vi "FPGAmain_5782_Fast_PID_v2.vi"() -> ()   [LabVIEW 2013]
uses:
  FPGA/DataMode.ctl
  FPGA/Input_5782/5782_states.ctl
  <vilib>/Platform/TimedLoop/XDataNode/timing_clust.ctl
  <vilib>/Platform/TimedLoop/XDataNode/nitl_modes.ctl
  <vilib>/Platform/TimedLoop/XDataNode/wakeup.ctl
  <vilib>/rvi/Emulation/niFpgaSctlEmulationGetInTimedLoop.vi
  <vilib>/rvi/Emulation/niFpgaEmulationReportErrorSimple.vi
  <vilib>/rvi/Emulation/niFpgaGetClockAttributes.vi
  <vilib>/rvi/eio/common/nirviEmuTemplateMethod_errors.vi
  <vilib>/rvi/Emulation/niFpgaCriticalErrorInLSC.vi
  <vilib>/rvi/DataTransferAndStorage/Register/Emulation/niFpgaRegisterEmulationFpgaImpl.vi
  <instcachedir>/0/niFpgaRegisterEmulationFpgaImpl_DCF4BC0110594B98B44A971D60CEEC4D.lvgen/niFpgaRegisterEmulationFpgaImpl_DCF4BC0110594B98B44A971D60CEEC4D_009.vi
  <vilib>/rvi/DataTransferAndStorage/Container/Common/niFpgaContainerGetUniqueNameForEmu.vi
  <vilib>/rvi/FIFO/Fifo_Resource/nirvififoEmulationReadFpgaImpl.vi
  <vilib>/rvi/interface/RandomDataEmulation/nirviRandomDataMultiElementFPGAFIFO.vi
  <instcachedir>/0/nirviRandomDataMultiElementFPGAFIFO_F2B80EDE0D7944A08478D8D26097D4DB.lvgen/nirviRandomDataMultiElementFPGAFIFO_F2B80EDE0D7944A08478D8D26097D4DB_005.vi
  <vilib>/rvi/interface/RandomDataEmulation/niFpgaRandomDataHandleErrors.vi
  <instcachedir>/0/niFpgaRegisterEmulationFpgaImpl_DCF4BC0110594B98B44A971D60CEEC4D.lvgen/niFpgaRegisterEmulationFpgaImpl_DCF4BC0110594B98B44A971D60CEEC4D_013.vi
  <vilib>/rvi/interface/RandomDataEmulation/nirviRandomDataFPGAFIFO.vi
  <instcachedir>/0/niFpgaRegisterEmulationFpgaImpl_DCF4BC0110594B98B44A971D60CEEC4D.lvgen/niFpgaRegisterEmulationFpgaImpl_DCF4BC0110594B98B44A971D60CEEC4D_003.vi
  <vilib>/rvi/FIFO/Fifo_Resource/nirvififoEmulationWriteFpgaImpl.vi
  <instcachedir>/0/niFpgaRegisterEmulationFpgaImpl_DCF4BC0110594B98B44A971D60CEEC4D.lvgen/niFpgaRegisterEmulationFpgaImpl_DCF4BC0110594B98B44A971D60CEEC4D_011.vi
  <instcachedir>/0/niFpgaRegisterEmulationFpgaImpl_DCF4BC0110594B98B44A971D60CEEC4D.lvgen/niFpgaRegisterEmulationFpgaImpl_DCF4BC0110594B98B44A971D60CEEC4D_012.vi
  <instcachedir>/0/niFpgaRegisterEmulationFpgaImpl_DCF4BC0110594B98B44A971D60CEEC4D.lvgen/niFpgaRegisterEmulationFpgaImpl_DCF4BC0110594B98B44A971D60CEEC4D_007.vi
  <instcachedir>/0/niFpgaRegisterEmulationFpgaImpl_DCF4BC0110594B98B44A971D60CEEC4D.lvgen/niFpgaRegisterEmulationFpgaImpl_DCF4BC0110594B98B44A971D60CEEC4D_008.vi
  <instcachedir>/0/niFpgaRegisterEmulationFpgaImpl_DCF4BC0110594B98B44A971D60CEEC4D.lvgen/niFpgaRegisterEmulationFpgaImpl_DCF4BC0110594B98B44A971D60CEEC4D_021.vi
  <instcachedir>/0/niFpgaRegisterEmulationFpgaImpl_DCF4BC0110594B98B44A971D60CEEC4D.lvgen/niFpgaRegisterEmulationFpgaImpl_DCF4BC0110594B98B44A971D60CEEC4D_020.vi
  <vilib>/Platform/TimedLoop/XDataNode/XDataNode.xnode
  <vilib>/eio/EIONode/EIONode.xnode
  <vilib>/rvi/DataTransferAndStorage/Container/XNode/niFpgaContainer.xnode
  <vilib>/rvi/DataTransferAndStorage/Register/Emulation/niFpgaRegisterEmulation.vi
  <vilib>/rvi/FIFO/Fifo_Resource/nirvififoEmulationRead.vi
  <vilib>/rvi/interface/RandomDataEmulation/nirviRandomDataFpgaMultiElementTemplate.vi
  <vilib>/rvi/interface/RandomDataEmulation/nirviRandomDataFpgaReadWriteTemplate.vi
  <vilib>/rvi/FIFO/Fifo_Resource/nirvififoEmulationWrite.vi
  <vilib>/Platform/TimedLoop/XDataNode/XDNodeRunTimeDep.lvlib
panel:
  in  "IO Module\\AO Data Sync":bool=TRUE
  in  "IO Module\\SPI Write Data":u16
  out "IO Module\\SPI Read Data":u8
  in  "IO Module\\SPI Read":bool
  in  "IO Module\\SPI Write":bool
  in  "IO Module\\SPI Address":u16
  in  "IO Module\\SPI Device":u8
  out "IO Module\\SPI Idle":bool
  in  "AM phase":fxp<+,64,64>
  in  "delay phase":fxp<+,64,64>
  in  "User Command Commit":bool
  in  "User Command":u8
  out "User Command Idle":bool
  out "User Command Status":u8
  in  "User Data 0":u8
  in  "User Data 1":u8
  out "PLL Locked":bool
  out "User Error":bool
  out "Configured?":bool
  in  "Continuous":bool
  in  "5782 record length":u16=4000 caption="Samples Per Trigger" min=1 step=1
  in  "Trigger Acquisition":bool
  out "IO Module\\Trigger Input":bool
  in  "Downsample":fxp<+,8,8>=1.0
  in  "new coeffs":bool
  in  "FIR coeffs":fxp<+/-,18,18>[](array[numeric])
  in  "CIC Gain":fxp<+/-,32,1>=0.00390625 format="%#_32g"
  in  "Acquisition running":bool
  in  "Phase output":fxp<+,64,64>[](array[numeric])=[0.0, 0.0, 0.0, 0.0]
  in  "Simulated phase 5782":fxp<+,64,64>[](array[numeric])=[0.0, 0.0]
  in  "Mode":T1
  in  "Phase 5782":fxp<+,64,64>[](array[numeric])=[0.0, 0.0]
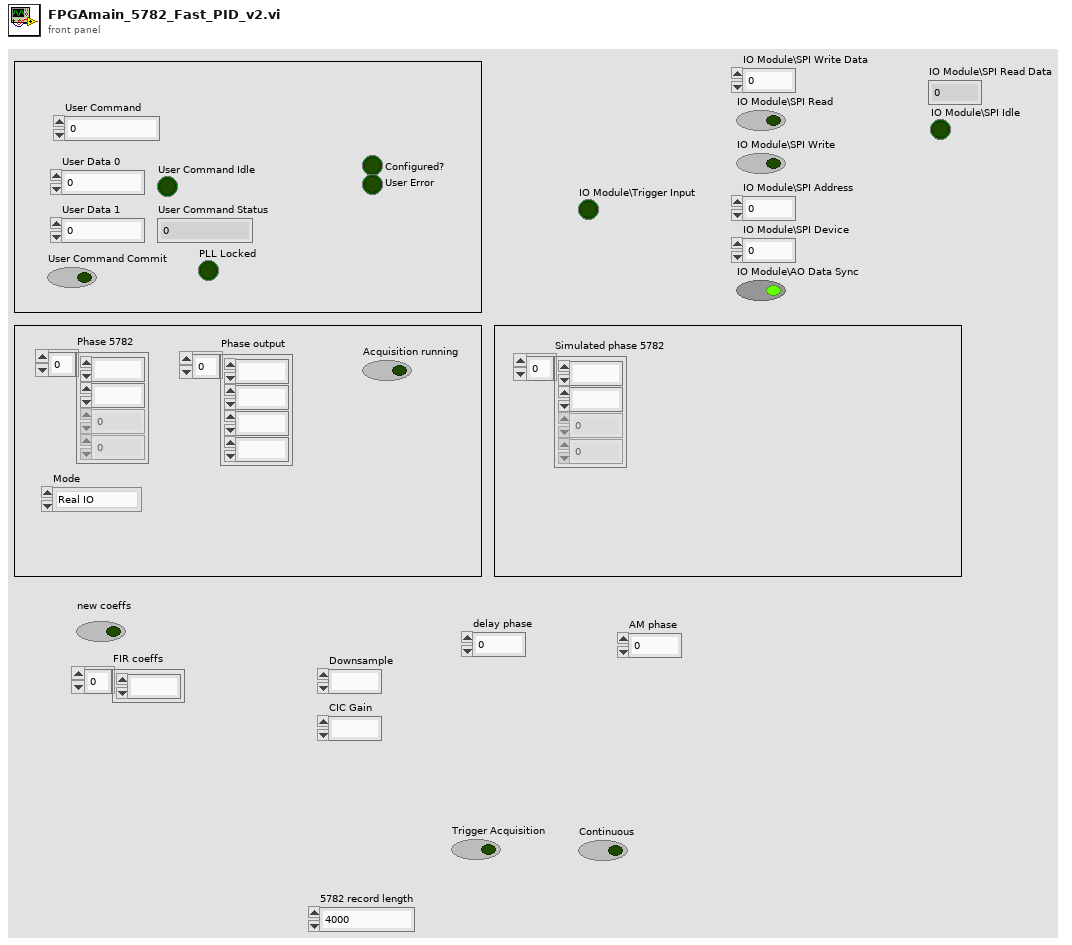
[diagram p1: front panel]
types:
  T1 = typedef "DataMode.ctl" = enum16{"Real IO", "Simulated"}
  T2 = typedef "5782_states.ctl" = enum8{"Wait for trigger", "Acquisition", "Send record length", "Quiet period"}
  T3 = typedef "XDNodeRunTimeDep.lvlib/timing_clust.ctl" = cluster{"Expected End [f-1]":u64, "Actual End [f-1]":u64, "Finished Late? [f-1]":bool, "Expected End [i-1]":u64, "Actual End [i-1]":u64, "Finished Late? [i-1]":bool, "Expected Start [i]":u64, "Actual Start [i]":u64, "Expected Start [f]":u64, "Actual Start [f]":u64, "Source Name":string, "Structure Name":string, "Period":i64, "Deadline":i64, "Offset":i64, "Start":i64, "Priority":i32, "Timeout":i32, "Mode":T4, "Wakeup Reason":T5, "Error":errorcluster, "Source Type":string, "Secondary Source Type":string, "Global End Time":u64, "Global Start Time":u64, "Frame Duration":u64, "Iteration Duration":u64, "Assigned CPU":i32, "I/O Scan Engine Mode":u32}
  T4 = typedef "XDNodeRunTimeDep.lvlib/nitl_modes.ctl" = enum32{"No Change", "Process missed periods, maintain original phase", "Discard missed periods, maintain original phase", "Process missed periods, ignore original phase", "Discard missed periods, ignore original phase"}
  T5 = typedef "XDNodeRunTimeDep.lvlib/wakeup.ctl" = enum32{"Normal", "Aborted", "Asynchronous wakeup", "Timing source error", "Timed loop error", "Timeout"}
  T6 = typedef "I16 array size 2.ctl" = i16[]
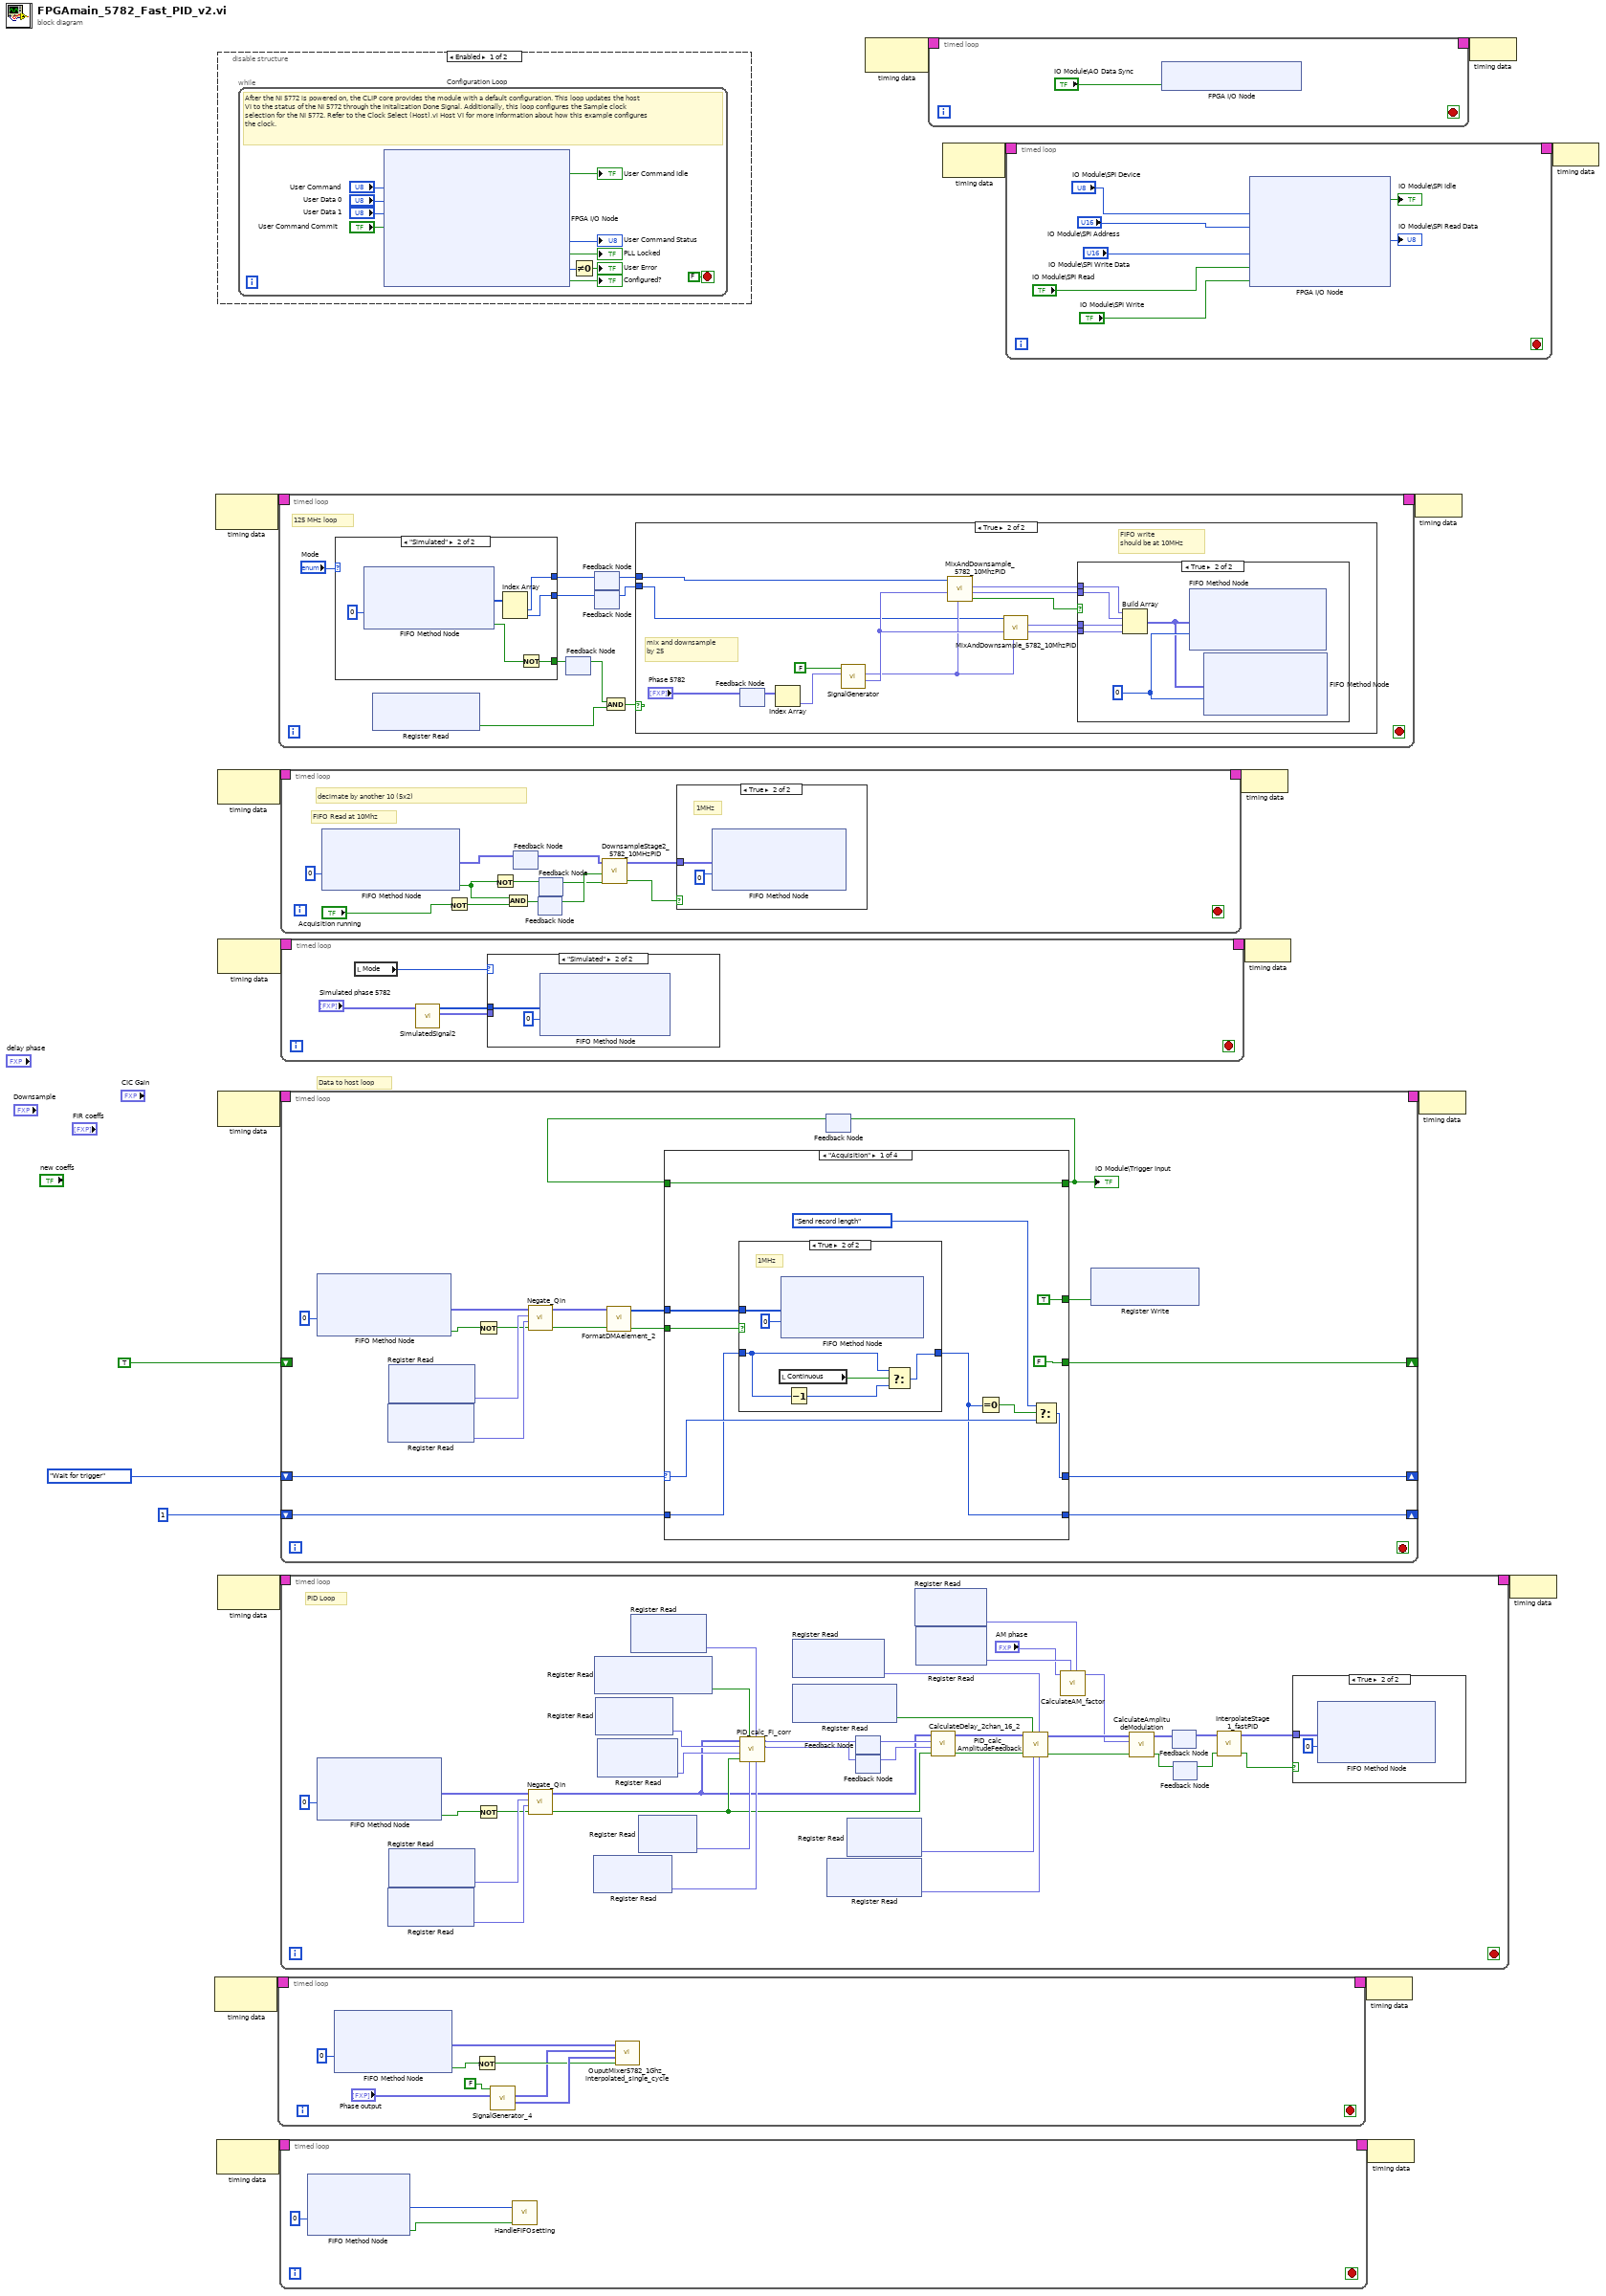
[diagram p0: block diagram]
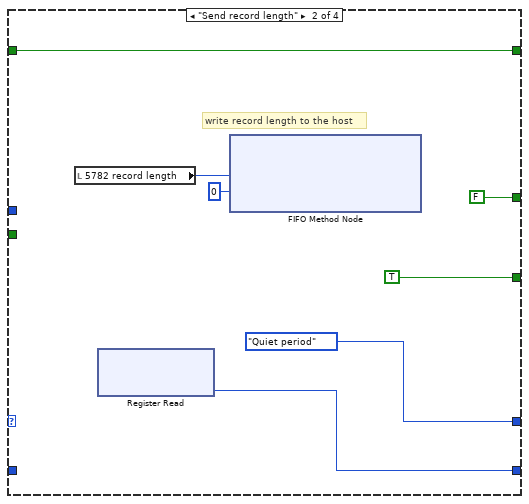
[diagram p3: hidden frame]
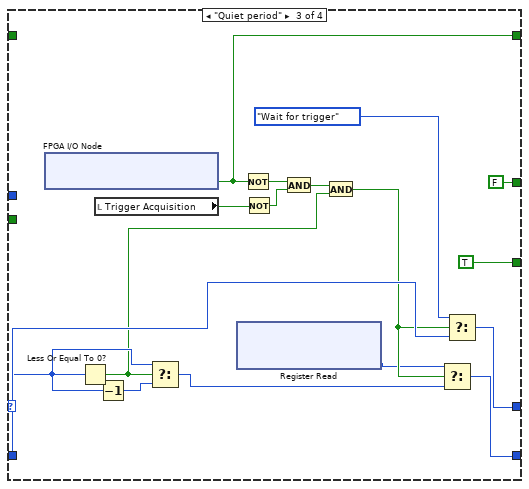
[diagram p4: hidden frame]
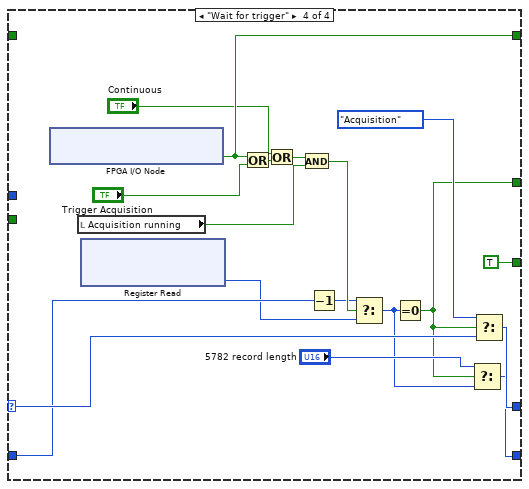
[diagram p5: hidden frame]
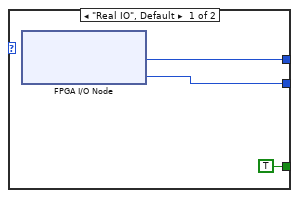
[diagram p11: hidden frame]
diagram:
  # "Data to host loop"
  n1 = node-c288() -> (w12:T3)  [unwired: 1 in]
  n2 = node-c288() -> (w19:T3)  [unwired: 1 in]
  n3 = node-c288() -> (w14:T3)  [unwired: 1 in]
  n4 = disable-structure shown="Enabled" {
    frame Enabled {
      n5 = while "Configuration Loop" {
        stop <- FALSE stop-if-true
        # "After the NI 5772 is powered on, the CLIP core provides the module with a default configuration. This loop updates the host VI to the status of the NI 5772 through the Initalization Done Signal. Additionally, this loop configures the Sample clock selection for the NI 5772. Refer to the Clock Select (Host).vi Host VI for more information about how this example configures the clock."
        n6 = xnode "FPGA I/O Node"("IO Module\\User Command"="User Command", "IO Module\\User Data 0"="User Data 0", "IO Module\\User Data 1"="User Data 1", "IO Module\\User Command Commit"="User Command Commit") -> ("IO Module\\User Command Idle"=→"User Command Idle":bool, "IO Module\\User Command Status"=→"User Command Status":u8, "IO Module\\PLL Locked"=→"PLL Locked":bool, "IO Module\\User Error"=w27:u8, "IO Module\\Initialization Done"=→"Configured?":bool)  [unwired: 9 in, 9 out]
        n7 = Not Equal To 0?(x=w27) -> (x != 0?=→"User Error":bool)
      }
    }
    frame Disabled {
    }
  }
  n8 = node-c288() -> (w4:T3)  [unwired: 1 in]
  n9 = node-c288() -> (w2:T3)  [unwired: 1 in]
  n10 = node-c288() -> (w6:T3)  [unwired: 1 in]
  n11 = node-c288() -> (w21:T3)  [unwired: 1 in]
  n12 = timed-loop {
    timing: w12 -> [_]
    timing-out: [_] -> w11
    stop <- _ stop-if-true
    n13 = xnode ("FIFO Method Node")("Timeout"=0) -> ("Element"=w35:fxp<+/-,16,14>[], "Timed Out?"=w39:bool)  [unwired: 1 in, 1 out]
    n14 = Not(x=w39) -> (.not. x?=w34:bool)
    n15 = call "SignalGenerator_4.vi"("Phase"="Phase output", "reset"=FALSE) -> ("Sine out"=w36:fxp<+/-,16,0>[], "Cosine out"=w33:fxp<+/-,16,0>[])  [unwired: 8 in]
    n16 = call "OuputMixer5782_1Ghz_interpolated_single_cycle.vi"("input valid"=w34, "Sine in"=w36, "Cosine in"=w33, "Data"=w35) -> ()  [unwired: 7 in, 1 out]
  }
  n17 = timed-loop {
    timing: w19 -> [_]
    timing-out: [_] -> w18
    stop <- _ stop-if-true
    # "125 MHz loop"
    n18 = case shown="\"Simulated\"" "Mode" {
      tunnel: [w73 w76] -> w49
      tunnel: [w72 w77] -> w47
      tunnel: [TRUE w74] -> w45
      frame "Real IO", Default {
        n19 = xnode "FPGA I/O Node"() -> ("IO Module\\AI 0"=w73:i16, "IO Module\\AI 1"=w72:i16)  [unwired: 2 in, 2 out]
      }
      frame "Simulated" {
        n20 = xnode ("FIFO Method Node")("Timeout"=0) -> ("Element"=w78:i16[], "Timed Out?"=w75:bool)  [unwired: 1 in, 1 out]
        n21 = Index Array(array=w78) -> (element #1=w76:i16, element #2=w77:i16)  [unwired: 2 in]
        n22 = Not(x=w75) -> (.not. x?=w74:bool)
      }
    }
    n23 = xnode ("Register Read")() -> ("Data"=w43:bool)  [unwired: 1 in, 1 out]
    n24 = feedback #1() -> (w44:bool)  [unwired: 1 in]
    n25 = feedback-in #1(w45) -> ()
    n26 = feedback #2() -> (w48:i16)  [unwired: 1 in]
    n27 = feedback-in #2(w49) -> ()
    n28 = feedback #3() -> (w46:i16)  [unwired: 1 in]
    n29 = feedback-in #3(w47) -> ()
    n30 = And(x=w44, y=w43) -> (x .and. y?=w50:bool)
    n31 = case shown="True" w50 {
      tunnel: w48 -> [_ w55]
      tunnel: w46 -> [_ w52]
      frame False {
      }
      frame True {
        # "FIFO write\nshould be at 10MHz"
        # "mix and downsample\nby 25"
        n32 = feedback #4() -> (w59:fxp<+,64,64>[])  [unwired: 1 in]
        n33 = feedback-in #4("Phase 5782") -> ()
        n34 = Index Array(array=w59) -> (element=w58:fxp<+,64,64>)  [unwired: 1 in]
        n35 = call "SignalGenerator.vi"("phase"=w58, "Reset"=FALSE) -> ("Cos"=w54:fxp<+/-,16,0>, "Sin"=w53:fxp<+/-,16,0>)  [unwired: 7 in, 1 out]
        n36 = call "MixAndDownsample_5782_10MhzPID.vi"("sin0"=w53, "cos0"=w54, "signal 0"=w55) -> ("data valid"=w62:bool, "Q out"=w63:fxp<+/-,16,14>, "I out"=w64:fxp<+/-,16,14>)  [unwired: 6 in]
        n37 = call "MixAndDownsample_5782_10MhzPID.vi"("sin0"=w53, "cos0"=w54, "signal 0"=w52) -> ("Q out"=w60:fxp<+/-,16,14>, "I out"=w61:fxp<+/-,16,14>)  [unwired: 6 in, 1 out]
        n38 = case shown="True" w62 {
          tunnel: w63 -> [_ w70]
          tunnel: w64 -> [_ w69]
          tunnel: w61 -> [_ w68]
          tunnel: w60 -> [_ w67]
          frame False {
          }
          frame True {
            w66 = 0 ("Timeout")
            n39 = Build Array(w69, w70, w68, w67) -> (w65:fxp<+/-,16,14>[])
            n40 = xnode ("FIFO Method Node")("Element"=w65, "Timeout"=w66) -> ()  [unwired: 1 in, 2 out]
            n41 = xnode ("FIFO Method Node")("Element"=w65, "Timeout"=w66) -> ()  [unwired: 1 in, 2 out]
          }
        }
      }
    }
  }
  n42 = timed-loop {
    timing: w14 -> [_]
    timing-out: [_] -> w13
    stop <- _ stop-if-true
    n43 = xnode ("FIFO Method Node")("Timeout"=0) -> ("Element"=w83:u64, "Timed Out?"=w82:bool)  [unwired: 1 in, 1 out]
    n44 = call "HandleFIFOsetting.vi"("timed out"=w82, "Value"=w83) -> ()  [unwired: 10 in]
  }
  n45 = timed-loop {
    timing: w4 -> [_]
    timing-out: [_] -> w3
    stop <- _ stop-if-true
    # "FIFO Read at 10Mhz"
    # "decimate by another 10 (5x2)"
    n46 = xnode ("FIFO Method Node")("Timeout"=0) -> ("Element"=w92:fxp<+/-,16,14>[], "Timed Out?"=w94:bool)  [unwired: 1 in, 1 out]
    n47 = Not(x="Acquisition running") -> (.not. x?=w95:bool)
    n48 = Not(x=w94) -> (.not. x?=w88:bool)
    n49 = And(x=w94, y=w95) -> (x .and. y?=w90:bool)
    n50 = feedback #5() -> (w91:fxp<+/-,16,14>[])  [unwired: 1 in]
    n51 = feedback-in #5(w92) -> ()
    n52 = feedback #6() -> (w89:bool)  [unwired: 1 in]
    n53 = feedback-in #6(w90) -> ()
    n54 = feedback #7() -> (w87:bool)  [unwired: 1 in]
    n55 = feedback-in #7(w88) -> ()
    n56 = call "DownsampleStage2_5782_10MHzPID.vi"("valid in"=w87, "reset"=w89, "Data in"=w91) -> ("valid out"=w96:bool, "data out"=w97:fxp<+/-,16,14>[])  [unwired: 7 in]
    n57 = case shown="True" w96 {
      tunnel: w97 -> [_ w99]
      frame False {
      }
      frame True {
        # "1MHz"
        n58 = xnode ("FIFO Method Node")("Element"=w99, "Timeout"=0) -> ()  [unwired: 1 in, 2 out]
      }
    }
  }
  n59 = timed-loop {
    timing: w2 -> [_]
    timing-out: [_] -> w1
    shift-right: [w118] -> _
    shift-left: 5782_states."Wait for trigger" ("5782 states") -> [w120]
    shift-right: [w117] -> _
    shift-left: u16 1 ("trigger samples") -> [w119]
    shift-right: [w112] -> _
    shift-left: TRUE -> [_]
    stop <- _ stop-if-true
    n60 = xnode ("FIFO Method Node")("Timeout"=0) -> ("Element"=w105:fxp<+/-,16,14>[], "Timed Out?"=w115:bool)  [unwired: 1 in, 1 out]
    n61 = xnode ("Register Read")() -> ("Data"=w107:fxp<+/-,16,14>)  [unwired: 1 in, 1 out]
    n62 = xnode ("Register Read")() -> ("Data"=w108:fxp<+/-,16,14>)  [unwired: 1 in, 1 out]
    n63 = Not(x=w115) -> (.not. x?=w106:bool)
    n64 = call "Negate_Qin.vi"("valid in"=w106, "DC offset chan 1"=w107, "DC offset chan 0"=w108, "Data in"=w105) -> ("valid out"=w103:bool, "Data out"=w104:fxp<+/-,16,14>[])  [unwired: 6 in]
    n65 = call "FormatDMAelement_2.vi"("valid in"=w103, "Data in"=w104) -> ("valid out"=w113:bool, "Element"=w114:u64[])  [unwired: 8 in]
    n66 = feedback #8() -> (w110:bool)  [unwired: 1 in]
    n67 = case shown="\"Acquisition\"" w120 {
      selector: w120 -> [w131 _ w161 w180]
      tunnel: w119 -> [w127 _ w149 w167]
      tunnel: [w130 5782_states."Quiet period" ("5782 states") w160 w179] -> w118
      tunnel: [w124 w139 w162 w178] -> w117
      tunnel: w114 -> [w125 _ _ _]
      tunnel: w113 -> [w126 _ _ _]
      tunnel: [FALSE TRUE TRUE TRUE] -> w112
      tunnel: [TRUE FALSE ("5782 triggered") FALSE ("5782 triggered") w171] -> w111
      tunnel: [w123 w140 w151 w170] -> w109
      tunnel: w110 -> [w123 w140 _ _]
      frame "Acquisition" {
        n68 = case shown="True" w126 {
          tunnel: w125 -> [_ w138]
          tunnel: [w132 w135] -> w124
          tunnel: w127 -> [w132 w133]
          frame False {
          }
          frame True {
            # "1MHz"
            n69 = local read "Continuous"() -> (w136:bool)
            n70 = xnode ("FIFO Method Node")("Element"=w138, "Timeout"=0) -> ()  [unwired: 1 in, 2 out]
            n71 = Decrement(x=w133) -> (x-1=w134:u16)
            n72 = Select(t=w133, s=w136, f=w134) -> (s? t:f=w135:u16)
          }
        }
        n73 = Equal To 0?(x=w124) -> (x = 0?=w128:bool)
        n74 = Select(t=5782_states."Send record length" ("5782 states"), s=w128, f=w131) -> (s? t:f=w130:T2)
      }
      frame "Send record length" {
        # "write record length to the host"
        n75 = local read "5782 record length"() -> (w142:u16)
        n76 = xnode ("Register Read")() -> ("Data"=w139:u16)  [unwired: 1 in, 1 out]
        n77 = xnode ("FIFO Method Node")("Element"=w142, "Timeout"=0) -> ()  [unwired: 1 in, 2 out]
      }
      frame "Quiet period" {
        n78 = xnode "FPGA I/O Node"() -> ("IO Module\\Trigger Input"=w151:bool)  [unwired: 1 in, 1 out]
        n79 = Less Or Equal To 0?(x=w149) -> (x <= 0?=w148:bool)
        n80 = local read "Trigger Acquisition"() -> (w157:bool)
        n81 = Decrement(x=w149) -> (x-1=w150:u16)
        n82 = Select(t=w149, s=w148, f=w150) -> (s? t:f=w147:u16)
        n83 = xnode ("Register Read")() -> ("Data"=w146:u16)  [unwired: 1 in, 1 out]
        n84 = Not(x=w151) -> (.not. x?=w156:bool)
        n85 = Not(x=w157) -> (.not. x?=w155:bool)
        n86 = And(x=w156, y=w155) -> (x .and. y?=w154:bool)
        n87 = And(x=w154, y=w148) -> (x .and. y?=w159:bool)
        n88 = Select(t=w146, s=w159, f=w147) -> (s? t:f=w162:u16)
        n89 = Select(t=5782_states."Wait for trigger" ("5782 states"), s=w159, f=w161) -> (s? t:f=w160:T2)
      }
      frame "Wait for trigger" {
        n90 = xnode "FPGA I/O Node"() -> ("IO Module\\Trigger Input"=w170:bool)  [unwired: 1 in, 1 out]
        n91 = local read "Acquisition running"() -> (w172:bool)
        n92 = xnode ("Register Read")() -> ("Data"=w163:u16)  [unwired: 1 in, 1 out]
        n93 = Or(x=w170, y="Trigger Acquisition") -> (x .or. y?=w166:bool)
        n94 = Or(x="Continuous", y=w166) -> (x .or. y?=w164:bool)
        n95 = And(x=w164, y=w172) -> (x .and. y?=w173:bool)
        n96 = Decrement(x=w167) -> (x-1=w168:u16)
        n97 = Select(t=w168, s=w173, f=w163) -> (s? t:f=w169:u16)
        n98 = Equal To 0?(x=w169) -> (x = 0?=w171:bool)
        n99 = Select(t="5782 record length", s=w171, f=w169) -> (s? t:f=w178:u16)
        n100 = Select(t=5782_states."Acquisition" ("5782 states"), s=w171, f=w180) -> (s? t:f=w179:T2)
      }
    }
    "IO Module\\Trigger Input" <- w109
    n101 = feedback-in #8(w109) -> ()
    n102 = xnode ("Register Write")("Data"=w111) -> ()  [unwired: 1 in, 1 out]
  }
  n103 = timed-loop {
    timing: w6 -> [_]
    timing-out: [_] -> w5
    stop <- _ stop-if-true
    # "PID Loop"
    n104 = xnode ("FIFO Method Node")("Timeout"=0) -> ("Element"=w206:fxp<+/-,16,14>[], "Timed Out?"=w217:bool)  [unwired: 1 in, 1 out]
    n105 = xnode ("Register Read")() -> ("Data"=w213:fxp<+/-,16,14>)  [unwired: 1 in, 1 out]
    n106 = xnode ("Register Read")() -> ("Data"=w214:fxp<+/-,16,14>)  [unwired: 1 in, 1 out]
    n107 = Not(x=w217) -> (.not. x?=w207:bool)
    n108 = call "Negate_Qin.vi"("valid in"=w207, "DC offset chan 1"=w213, "DC offset chan 0"=w214, "Data in"=w206) -> ("valid out"=w197:bool, "Data out"=w196:fxp<+/-,16,14>[])  [unwired: 6 in]
    n109 = xnode ("Register Read")() -> ("Data"=w204:fxp<+/-,32,4>)  [unwired: 1 in, 1 out]
    n110 = xnode ("Register Read")() -> ("Data"=w201:bool)  [unwired: 1 in, 1 out]
    n111 = xnode ("Register Read")() -> ("Data"=w202:fxp<+/-,32,4>)  [unwired: 1 in, 1 out]
    n112 = xnode ("Register Read")() -> ("Data"=w203:fxp<+/-,32,4>)  [unwired: 1 in, 1 out]
    n113 = xnode ("Register Read")() -> ("Data"=w200:fxp<+/-,32,4>)  [unwired: 1 in, 1 out]
    n114 = xnode ("Register Read")() -> ("Data"=w205:fxp<+/-,32,4>)  [unwired: 1 in, 1 out]
    n115 = call "PID_calc_Fi_corr.vi"("Kd/Tau"=w204, "Ki*Tau"=w200, "Kp"=w205, "Enabled"=w201, "input valid"=w197, "Fi_delta"=w203, "Fi_start"=w202, "Data in"=w196) -> ("cos_fi_korr"=w198:fxp<+/-,16,2>, "sin fi_korr"=w199:fxp<+/-,16,2>)  [unwired: 2 out]
    n116 = xnode ("Register Read")() -> ("Data"=w211:bool)  [unwired: 1 in, 1 out]
    n117 = xnode ("Register Read")() -> ("Data"=w208:fxp<+/-,32,6>)  [unwired: 1 in, 1 out]
    n118 = xnode ("Register Read")() -> ("Data"=w209:fxp<+/-,32,6>)  [unwired: 1 in, 1 out]
    n119 = xnode ("Register Read")() -> ("Data"=w210:fxp<+/-,32,6>)  [unwired: 1 in, 1 out]
    n120 = feedback-in #9(w199) -> ()
    n121 = feedback #9() -> (w216:fxp<+/-,16,2>)  [unwired: 1 in]
    n122 = feedback #10() -> (w215:fxp<+/-,16,2>)  [unwired: 1 in]
    n123 = feedback-in #10(w198) -> ()
    n124 = xnode ("Register Read")() -> ("Data"=w190:fxp<+/-,16,2>)  [unwired: 1 in, 1 out]
    n125 = xnode ("Register Read")() -> ("Data"=w191:fxp<+/-,16,2>)  [unwired: 1 in, 1 out]
    n126 = call "CalculateDelay_2chan_16_2.vi"("input valid"=w197, "cos_fi"=w215, "sin fi"=w216, "Data in"=w196) -> ("output valid"=w195:bool, "Data out"=w212:fxp<+/-,16,14>[])  [unwired: 6 in]
    n127 = call "PID_calc_AmplitudeFeedback.vi"("Kd/Tau"=w209, "Ki*Tau"=w208, "Kp"=w210, "Enabled"=w211, "input valid"=w195, "Data in"=w212) -> ("output valid"=w192:bool, "data out"=w194:fxp<+/-,16,14>[])  [unwired: 2 in, 2 out]
    n128 = call "CalculateAM_factor.vi"("b_am"=w190, "a_am"=w191, "AM phase"="AM phase") -> ("AM_factor"=w189:fxp<+/-,16,2>)  [unwired: 7 in, 1 out]
    n129 = call "CalculateAmplitudeModulation.vi"("input valid"=w192, "AM_factor"=w189, "Data in"=w194) -> ("output valid"=w188:bool, "Data out"=w193:fxp<+/-,16,14>[])  [unwired: 7 in]
    n130 = feedback #11() -> (w186:fxp<+/-,16,14>[])  [unwired: 1 in]
    n131 = feedback-in #11(w193) -> ()
    n132 = feedback #12() -> (w184:bool)  [unwired: 1 in]
    n133 = feedback-in #12(w188) -> ()
    n134 = call "InterpolateStage1_fastPID.vi"("valid in"=w184, "Data in"=w186) -> ("valid out"=w183:bool, "Data out"=w185:fxp<+/-,16,14>[])  [unwired: 8 in]
    n135 = case shown="True" w183 {
      tunnel: w185 -> [_ w219]
      frame False {
      }
      frame True {
        n136 = xnode ("FIFO Method Node")("Element"=w219, "Timeout"=0) -> ()  [unwired: 1 in, 2 out]
      }
    }
  }
  n137 = timed-loop {
    timing: w21 -> [_]
    timing-out: [_] -> w20
    stop <- _ stop-if-true
    n138 = local read "Mode"() -> (w226:T1)
    n139 = call "SimulatedSignal2.vi"("Phase"="Simulated phase 5782") -> ("dummy do not use"=w223:fxp<+/-,16,0>[], "output"=w225:T6)  [unwired: 9 in]
    n140 = case shown="\"Simulated\"" w226 {
      tunnel: w225 -> [_ w227]
      tunnel: w223 -> [_ _]
      frame "Real IO", Default {
      }
      frame "Simulated" {
        n141 = xnode ("FIFO Method Node")("Element"=w227, "Timeout"=0) -> ()  [unwired: 1 in, 2 out]
      }
    }
  }
  n142 = node-c288() -> (w8:T3)  [unwired: 1 in]
  n143 = timed-loop {
    timing: w8 -> [_]
    timing-out: [_] -> w7
    stop <- _ stop-if-true
    n144 = xnode "FPGA I/O Node"("IO Module\\AO Data Sync"="IO Module\\AO Data Sync") -> ()  [unwired: 1 in, 1 out]
  }
  n145 = node-c288() -> (w10:T3)  [unwired: 1 in]
  n146 = timed-loop {
    timing: w10 -> [_]
    timing-out: [_] -> w9
    stop <- _ stop-if-true
    n147 = xnode "FPGA I/O Node"("IO Module\\SPI Device"="IO Module\\SPI Device", "IO Module\\SPI Address"="IO Module\\SPI Address", "IO Module\\SPI Write Data"="IO Module\\SPI Write Data", "IO Module\\SPI Read"="IO Module\\SPI Read", "IO Module\\SPI Write"="IO Module\\SPI Write") -> ("IO Module\\SPI Idle"=→"IO Module\\SPI Idle":bool, "IO Module\\SPI Read Data"=→"IO Module\\SPI Read Data":u8)  [unwired: 7 in, 7 out]
  }
  n148 = node-c288(w3) -> ()
  n149 = node-c288(w20) -> ()
  n150 = node-c288(w11) -> ()
  n151 = node-c288(w13) -> ()
  n152 = node-c288(w18) -> ()
  n153 = node-c288(w1) -> ()
  n154 = node-c288(w7) -> ()
  n155 = node-c288(w5) -> ()
  n156 = node-c288(w9) -> ()
